vi "Find Nearest Edge.vi"(7 "Pane Coordinates":T3, 8 "error in (no error)":errorcluster, 11 "Pane Object Position in":refnum<class "Pane Object Position.lvclass">) -> (0 "error out":errorcluster, 1 "Direction":T1, 2 "Nearest Side":T2=enum."Top", 3 "Pane Object Position out":refnum<class "Pane Object Position.lvclass">)   [LabVIEW 2018, in "Pane Object Position.lvclass"]
uses:
  Pane Object Position.lvclass
  Object Coordinates.ctl
  Pane Position Enum.ctl
  Direction Ctl.ctl
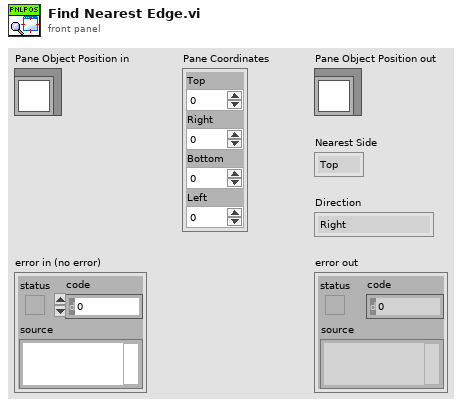
[diagram p1: front panel]
types:
  T1 = typedef "Direction Ctl.ctl" = enum16{"Right", "Left", "Up", "Down"}
  T2 = typedef "Pane Object Position.lvclass/Pane Position Enum.ctl" = enum16{"Indeterminate", "Top", "Right", "Top Right", "Bottom", "5", "Bottom Right", "7", "Left", "Top Left", "10", "11", "Bottom Left"}
  T3 = typedef "Pane Object Position.lvclass/Object Coordinates.ctl" = cluster{"Top":i32, "Right":i32, "Bottom":i32, "Left":i32}
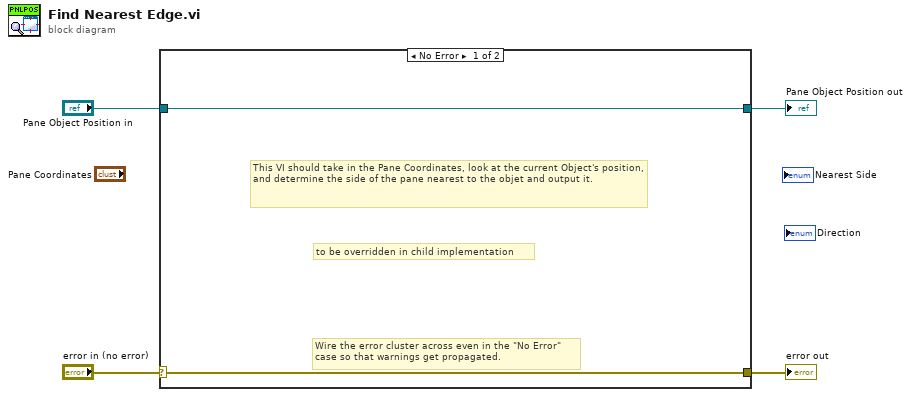
[diagram p0: block diagram]
diagram:
  n1 = case shown="No Error" "error in (no error)" {
    selector: "error in (no error)" -> [w5 w8]
    tunnel: [w5 w8] -> w3
    tunnel: [w6 w7] -> w1
    tunnel: "Pane Object Position in" -> [w6 w7]
    frame No Error {
      # "This VI should take in the Pane Coordinates, look at the current Object's position, and determine the side of the pane nearest to the objet and output it."
      # "to be overridden in child implementation"
      # "Wire the error cluster across even in the \"No Error\"\ncase so that warnings get propagated."
    }
    frame Error {
    }
  }
  "error out" <- w3
  "Pane Object Position out" <- w1
